vi "S2C_XML_CreateEvent.vi"(8 "Error In":errorcluster) -> (0 "Error Out":errorcluster)   [LabVIEW 2015]
uses:
  S2C_XML_Globals.vi
  <vilib>/xml/Close Reference(Node).vi
  <resource>/objmgr/DOMUserDefRef.rc
  <vilib>/xml/NI_XML.lvlib
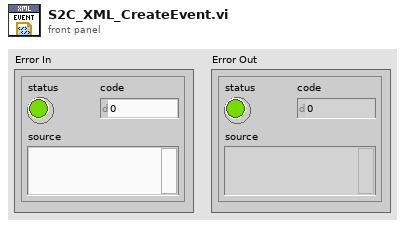
[diagram p1: front panel]
types:
  T1 = cluster{"EventName":string, "ProcessName":string, "ProductLine":string, "EventStatus":string, "EventStart":string, "EventStop":string, "Station":string, "OperatorName":string, "Location":string}
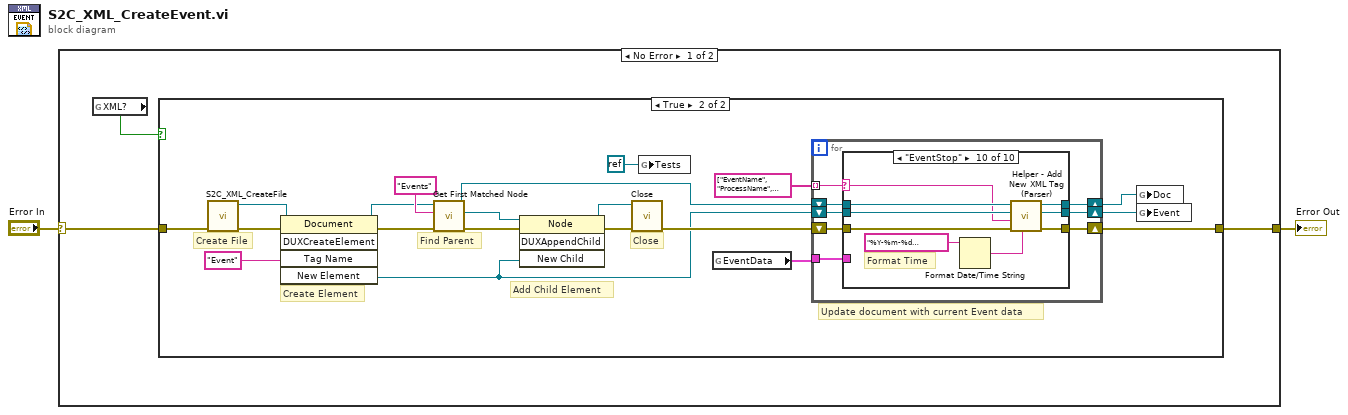
[diagram p0: block diagram]
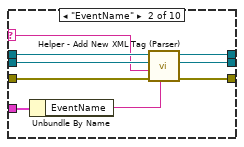
[diagram p4: hidden frame]
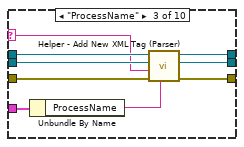
[diagram p5: hidden frame]
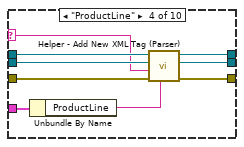
[diagram p6: hidden frame]
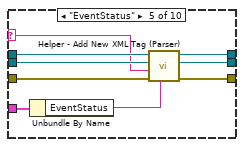
[diagram p7: hidden frame]
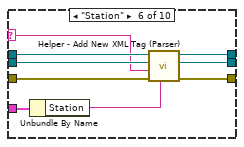
[diagram p8: hidden frame]
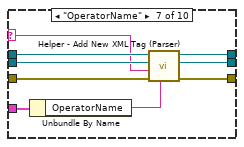
[diagram p9: hidden frame]
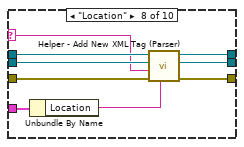
[diagram p10: hidden frame]
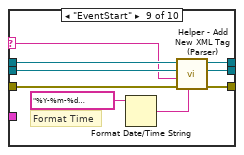
[diagram p11: hidden frame]
diagram:
  n1 = case shown="No Error" "Error In" {
    selector: "Error In" -> [w5 w119]
    tunnel: [w4 w119] -> w2
    frame No Error {
      n2 = global read "S2C_XML_Globals.vi" "XML?"() -> (w3:bool)
      n3 = case shown="True" w3 {
        tunnel: w5 -> [w6 w9]
        tunnel: [w6 w11] -> w4
        frame False {
          # "The XML Output is currently disabled"
        }
        frame True {
          # "Create File"
          # "Update document with current Event data"
          # "Close"
          # "Add Child Element"
          # "Find Parent"
          # "Create Element"
          n4 = call "S2C_XML_CreateFile.vi"("Error In"=w9) -> ("Error Out"=w8:errorcluster, "DocRef"=w7:refnum<k20>)  [unwired: 9 in]
          n5 = invoke class="Document" method="DUXCreateElement"(reference=w7, error in=w8, "Tag Name"="Event") -> (reference out=w21:refnum<k20>, error out=w22:errorcluster, "New Element"=w14:refnum<k20>)  [unwired: 2 in, 2 out]
          n6 = call <vilib>:"Get First Matched Node.vi"("error in (no error)"=w22, "XPath expression"="Events", "node in"=w21) -> ("error out"=w25:errorcluster, "node result"=w24:refnum<k20>, "node out"=w15:refnum<k20>)  [unwired: 6 in]
          n7 = invoke class="Node" method="DUXAppendChild"(reference=w24, error in=w25, "New Child"=w14) -> (reference out=w19:refnum<k20>, error out=w20:errorcluster)  [unwired: 1 in, 2 out]
          n8 = call-poly <vilib>:"Close.vi"("error in (no error)"=w20, "node"=w19) -> ("error out"=w17:errorcluster)  [unwired: 7 in]
          n9 = global write "S2C_XML_Globals.vi" "Tests"(refnum<k0> refnum) -> ()
          n10 = global read "S2C_XML_Globals.vi" "EventData"() -> (w10:T1)
          n11 = for {
            tunnel: string[] ["EventName", "ProcessName", "ProductLine", "EventStatus", "EventStart", "EventStop", "Station", "OperatorName", "Location"] -> [w33] mode=indexing
            shift-right: [w27] -> w13
            shift-left: w15 -> [w32]
            shift-right: [w28] -> w12
            shift-left: w14 -> [w31]
            shift-right: [w29] -> w11
            shift-left: w17 -> [w34]
            tunnel: w10 -> [w30]
            n12 = case shown="\"EventStop\"" w33 {
              selector: w33 -> [_ w39 w48 w57 w66 w75 w84 w93 w103 w112]
              tunnel: w34 -> [w35 w45 w54 w63 w72 w81 w90 w99 w109 w118]
              tunnel: w32 -> [w37 w42 w51 w60 w69 w78 w87 w96 w106 w115]
              tunnel: [w37 w41 w50 w59 w68 w77 w86 w95 w105 w114] -> w27
              tunnel: w31 -> [w36 w43 w52 w61 w70 w79 w88 w97 w107 w116]
              tunnel: [w36 w40 w49 w58 w67 w76 w85 w94 w104 w113] -> w28
              tunnel: [w35 w44 w53 w62 w71 w80 w89 w98 w108 w117] -> w29
              tunnel: w30 -> [_ w46 w55 w64 w73 w82 w91 w100 _ _]
              frame "Unknown", Default {
              }
              frame "EventName" {
                n13 = Unbundle By Name(w46) -> ("EventName"=w38:string)
                n14 = call "Helper - Add New XML Tag (Parser).vi"("Tag Data"=w38, "error in (no error)"=w45, "Tag Name"=w39, "Owning Element"=w43, "DOM document"=w42) -> ("error out"=w44:errorcluster, "dup Owning Element"=w40:refnum<k20>, "dup DOM document"=w41:refnum<k20>)  [unwired: 4 in]
              }
              frame "ProcessName" {
                n15 = Unbundle By Name(w55) -> ("ProcessName"=w47:string)
                n16 = call "Helper - Add New XML Tag (Parser).vi"("Tag Data"=w47, "error in (no error)"=w54, "Tag Name"=w48, "Owning Element"=w52, "DOM document"=w51) -> ("error out"=w53:errorcluster, "dup Owning Element"=w49:refnum<k20>, "dup DOM document"=w50:refnum<k20>)  [unwired: 4 in]
              }
              frame "ProductLine" {
                n17 = Unbundle By Name(w64) -> ("ProductLine"=w56:string)
                n18 = call "Helper - Add New XML Tag (Parser).vi"("Tag Data"=w56, "error in (no error)"=w63, "Tag Name"=w57, "Owning Element"=w61, "DOM document"=w60) -> ("error out"=w62:errorcluster, "dup Owning Element"=w58:refnum<k20>, "dup DOM document"=w59:refnum<k20>)  [unwired: 4 in]
              }
              frame "EventStatus" {
                n19 = Unbundle By Name(w73) -> ("EventStatus"=w65:string)
                n20 = call "Helper - Add New XML Tag (Parser).vi"("Tag Data"=w65, "error in (no error)"=w72, "Tag Name"=w66, "Owning Element"=w70, "DOM document"=w69) -> ("error out"=w71:errorcluster, "dup Owning Element"=w67:refnum<k20>, "dup DOM document"=w68:refnum<k20>)  [unwired: 4 in]
              }
              frame "Station" {
                n21 = Unbundle By Name(w82) -> ("Station"=w74:string)
                n22 = call "Helper - Add New XML Tag (Parser).vi"("Tag Data"=w74, "error in (no error)"=w81, "Tag Name"=w75, "Owning Element"=w79, "DOM document"=w78) -> ("error out"=w80:errorcluster, "dup Owning Element"=w76:refnum<k20>, "dup DOM document"=w77:refnum<k20>)  [unwired: 4 in]
              }
              frame "OperatorName" {
                n23 = Unbundle By Name(w91) -> ("OperatorName"=w83:string)
                n24 = call "Helper - Add New XML Tag (Parser).vi"("Tag Data"=w83, "error in (no error)"=w90, "Tag Name"=w84, "Owning Element"=w88, "DOM document"=w87) -> ("error out"=w89:errorcluster, "dup Owning Element"=w85:refnum<k20>, "dup DOM document"=w86:refnum<k20>)  [unwired: 4 in]
              }
              frame "Location" {
                n25 = Unbundle By Name(w100) -> ("Location"=w92:string)
                n26 = call "Helper - Add New XML Tag (Parser).vi"("Tag Data"=w92, "error in (no error)"=w99, "Tag Name"=w93, "Owning Element"=w97, "DOM document"=w96) -> ("error out"=w98:errorcluster, "dup Owning Element"=w94:refnum<k20>, "dup DOM document"=w95:refnum<k20>)  [unwired: 4 in]
              }
              frame "EventStart" {
                # "Format Time"
                n27 = Format Date/Time String(time format string (%c)="%Y-%m-%d %H:%M:%S%3u") -> (date/time string=w101:string)  [unwired: 2 in]
                n28 = call "Helper - Add New XML Tag (Parser).vi"("Tag Data"=w101, "error in (no error)"=w109, "Tag Name"=w103, "Owning Element"=w107, "DOM document"=w106) -> ("error out"=w108:errorcluster, "dup Owning Element"=w104:refnum<k20>, "dup DOM document"=w105:refnum<k20>)  [unwired: 4 in]
              }
              frame "EventStop" {
                # "Format Time"
                n29 = Format Date/Time String(time format string (%c)="%Y-%m-%d %H:%M:%S%3u") -> (date/time string=w110:string)  [unwired: 2 in]
                n30 = call "Helper - Add New XML Tag (Parser).vi"("Tag Data"=w110, "error in (no error)"=w118, "Tag Name"=w112, "Owning Element"=w116, "DOM document"=w115) -> ("error out"=w117:errorcluster, "dup Owning Element"=w113:refnum<k20>, "dup DOM document"=w114:refnum<k20>)  [unwired: 4 in]
              }
            }
          }
          n31 = global write "S2C_XML_Globals.vi" "Doc"(w13) -> ()
          n32 = global write "S2C_XML_Globals.vi" "Event"(w12) -> ()
        }
      }
    }
    frame Error {
    }
  }
  "Error Out" <- w2
